vi "Get points on line.vi"(10 "Stop":cluster{"X":i32, "Y":i32}, 11 "Start":cluster{"X":i32, "Y":i32}) -> (3 "Line":cluster{"X":i32, "Y":i32}[](array[cluster]))   [LabVIEW 2021]
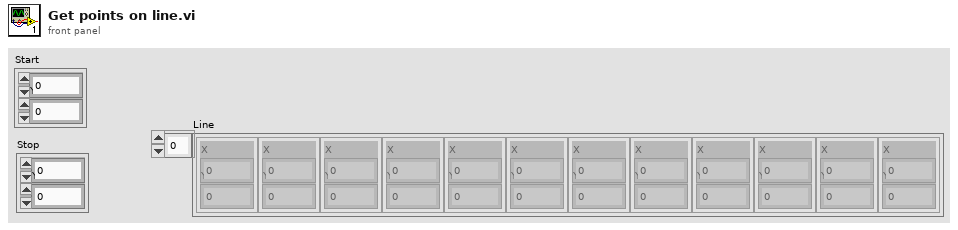
[diagram p1: front panel]
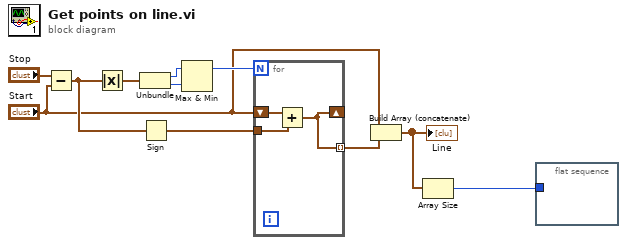
[diagram p0: block diagram]
diagram:
  n1 = Subtract(x="Stop", y="Start") -> (x-y=w8:cluster{"X":i32, "Y":i32})
  n2 = Absolute Value(x=w8) -> (abs(x)=w1:cluster{"X":i32, "Y":i32})
  n3 = Unbundle(w1) -> ("X"=w11:i32, "Y"=w10:i32)
  n4 = Sign(1:w8) -> (0:w6:cluster{"X":i32, "Y":i32})
  n5 = Max & Min(x=w11, y=w10) -> (max(x,y)=w9:i32)  [unwired: 1 out]
  n6 = for {
    N: w9 -> [_]
    tunnel: w6 -> [w14]
    tunnel: [w12] -> w4 mode=indexing
    shift-right: [w12] -> _
    shift-left: "Start" -> [w13]
    n7 = Add(x=w13, y=w14) -> (x+y=w12:cluster{"X":i32, "Y":i32})
  }
  n8 = Build Array (concatenate)("Start", w4) -> (w3:cluster{"X":i32, "Y":i32}[])
  "Line" <- w3
  n9 = Array Size(array=w3) -> (size(s)=w2:i32)
  n10 = flat-sequence {
    tunnel: w2 -> [_]
    frame #0 {
    }
  }
